vi "P5YL0.vi"() -> ()   [LabVIEW 2020]
panel:
  in  "Y 4":i32
  in  "X 3":i32
  out "Numeric 2":i32
  out "Numeric":i32
  out "Array 2":i32[](array[numeric])
  out "Array":i32[](array[numeric])
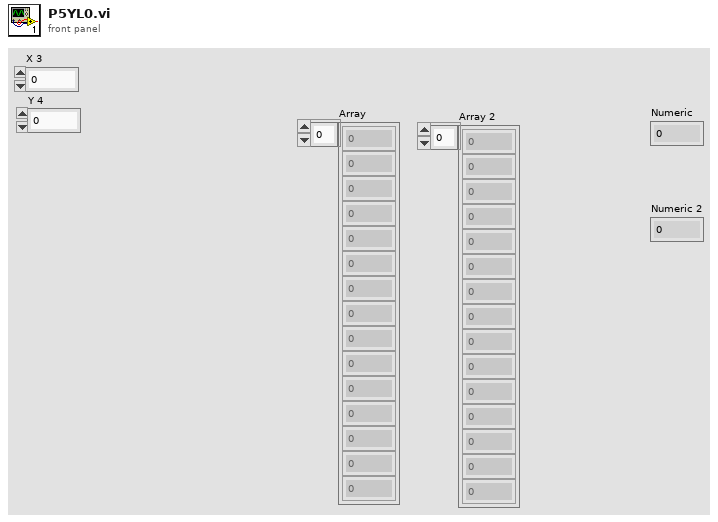
[diagram p1: front panel]
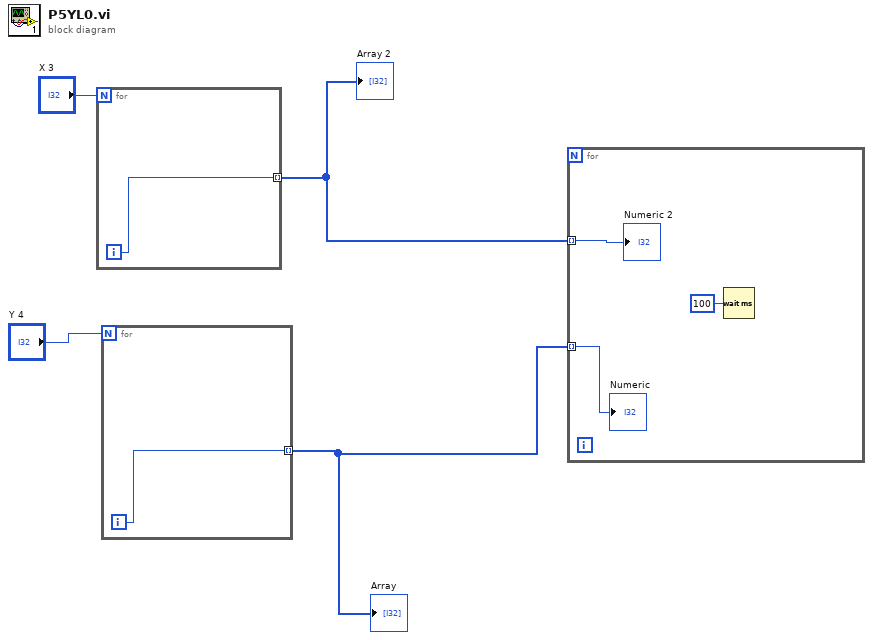
[diagram p0: block diagram]
diagram:
  n1 = for {
    N: "X 3" -> [_]
    tunnel: [w5] -> w3 mode=indexing
    i -> [w5]
  }
  "Array 2" <- w3
  n2 = for {
    N: "Y 4" -> [_]
    tunnel: [w6] -> w4 mode=indexing
    i -> [w6]
  }
  "Array" <- w4
  n3 = for {
    tunnel: w4 -> [w9] mode=indexing
    tunnel: w3 -> [w8] mode=indexing
    n4 = Wait (ms)(milliseconds to wait=u32 100) -> ()  [unwired: 1 out]
    "Numeric" <- w9
    "Numeric 2" <- w8
  }
